vi "_ReadInstruction.vi"(7 "Instructions":refnum<k21>, 8 "error in (no error)":errorcluster, 9 "Length":u8, 10 "FIFO In":refnum<k21>, 11 "MPU in":refnum<class "MPU.lvclass">) -> (0 "error out":errorcluster, 3 "MPU out":refnum<class "MPU.lvclass">)   [LabVIEW 2018, in "Modbus_Processing_Unit.lvlib" / "MPU.lvclass"]
uses:
  MPU.lvclass
  MPU.lvclass/MPU.ctl
  <vilib>/rvi/DataTransferAndStorage/Container/Common/niFpgaContainerExecOnDevCompGetState.vi
  <vilib>/rvi/Emulation/niFpgaEmulationIsFPGAContextNoSignature.vi
  <vilib>/rvi/Emulation/niFpgaSctlEmulationGetInTimedLoop.vi
  <vilib>/rvi/errors/niFpgaSetErrorForExecOnDevCompSimple.vi
  <vilib>/rvi/eio/common/nirviEmuReportErrorAndStop.vi
  <vilib>/rvi/DataTransferAndStorage/Container/Common/niFpgaContainerGetUniqueNameForEmu.vi
  <vilib>/rvi/FIFO/Fifo_Resource/nirvififoEmulationSetSize.vi
  <vilib>/rvi/FIFO/Fifo_Resource/nirviFifoEmulationQueueMgr.vi
  <instcachedir>/0/nirviFifoEmulationQueueMgr_E5CAEC123FF24DC58D834DCA3CDAA9B5.lvgen/nirviFifoEmulationQueueMgr_E5CAEC123FF24DC58D834DCA3CDAA9B5_001.vi
  <vilib>/rvi/FIFO/Fifo_Resource/nirvififoEmulationDetermineInputValidOut.vi
  <vilib>/rvi/FIFO/Fifo_Resource/nirvififoEmulationCreateLock.vi
  <vilib>/rvi/Emulation/niFpgaProcessEmulError.vi
  <vilib>/rvi/FIFO/Fifo_Resource/nirvififoEmulationObtainLock.vi
  <vilib>/rvi/FIFO/Fifo_Resource/nirvififoEmulationReleaseLock.vi
  <vilib>/rvi/occurrence/nirviWaitOnOccurrenceBase.vi
  <vilib>/rvi/errors/nirviReportUnexpectedCaseInternalError.vi
  <vilib>/rvi/errors/nirviReportUnexpectedCaseInternalError (U32).vi
  <vilib>/Utility/error.llb/Clear Errors.vi
  <vilib>/rvi/interface/RandomDataEmulation/niFpgaRandomDataHandleErrors.vi
  <vilib>/rvi/Memory/Memory_Emulation/niFpgaMemoryEmulationCacheClearOnFirstRun.vi
  <vilib>/rvi/Memory/Memory_Emulation/nirvimemoryEmulationManagerCache_MakeExclusive.vi
  <vilib>/rvi/Memory/Memory_Emulation/niFpgaMemoryEmulationValidateCache.vi
  <vilib>/rvi/Memory/Memory_Emulation/nirvimemoryEmulationManagerCache_InsertValue.vi
  <vilib>/rvi/Memory/Memory_Emulation/nirvimemoryEmulationManagerCache_ReleaseExclusive.vi
  <vilib>/rvi/Memory/Memory_Emulation/nirvimemoryEmulationManagerCache_GetValue.vi
  <vilib>/rvi/Memory/Memory_Emulation/nirvimemoryEmulationManagerCache_SetValue.vi
  <vilib>/rvi/Emulation/niFpgaSctlEmulationResourceMgr.vi
  <vilib>/rvi/DataTransferAndStorage/Container/XNode/niFpgaContainer.xnode
  <vilib>/rvi/FIFO/Fifo_Resource/niFpgaFifoEmulationRefIn.vi
  <vilib>/rvi/Memory/Memory_Emulation/niFpgaMemoryEmulationRefIn.vi
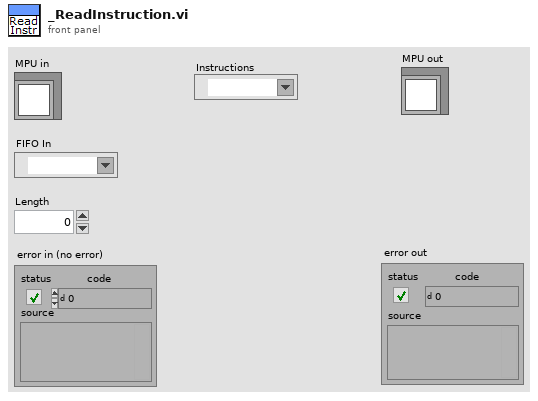
[diagram p1: front panel]
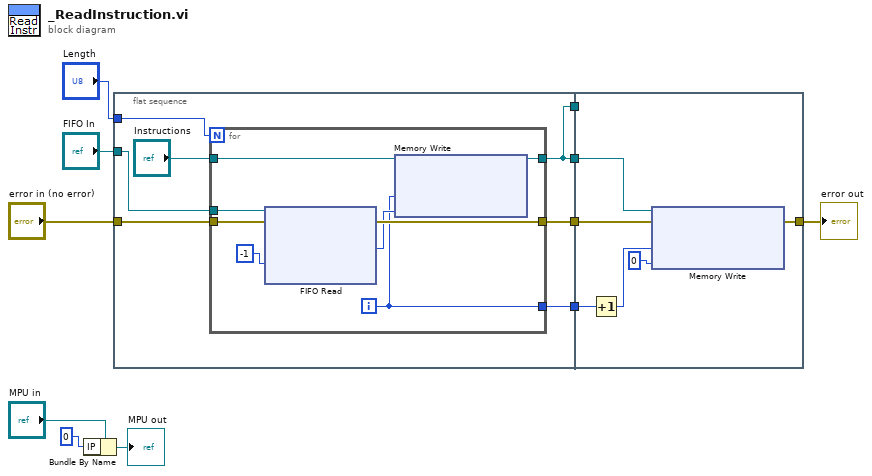
[diagram p0: block diagram]
diagram:
  n1 = Bundle By Name(cluster="MPU in", "IP"=i16 0) -> (→"MPU out":refnum<class "MPU.lvclass">)
  n2 = flat-sequence {
    tunnel: "Length" -> [w16]
    tunnel: "error in (no error)" -> [w18]
    tunnel: [w17] -> w11
    tunnel: [w15] -> w10
    tunnel: "FIFO In" -> [w14]
    tunnel: [w12] -> w2
    tunnel: [w12] -> w1
    tunnel: [w29] -> w4
    tunnel: w11 -> [w30]
    tunnel: w10 -> [w32]
    tunnel: w2 -> [_]
    tunnel: w1 -> [w31]
    frame #0 {
      n3 = for {
        N: w16 -> [_]
        tunnel: [w19] -> w15
        tunnel: w14 -> [w23]
        tunnel: w18 -> [w26]
        tunnel: [w25] -> w17
        tunnel: [w22] -> w12
        tunnel: "Instructions" -> [w21]
        i -> [w19]
        n4 = xnode ("FIFO Read")("Timeout"=-1, "error in (no error)"=w26, "FIFO In"=w23) -> ("Element"=w20:u8, "error out"=w25:errorcluster)  [unwired: 2 out]
        n5 = xnode ("Memory Write")("Address"=w19, "Data"=w20, "Memory In"=w21) -> ("Memory Out"=w22:refnum<k21>)
      }
    }
    frame #1 {
      n6 = Increment(x=w32) -> (x+1=w28:i32)
      n7 = xnode ("Memory Write")("Address"=w28, "Data"=u8 0, "error in (no error)"=w30, "Memory In"=w31) -> ("error out"=w29:errorcluster)  [unwired: 1 out]
    }
  }
  "error out" <- w4
